vi "Digital_Input_32Channels.vi"(1 "IO":T1={"DI 0"="Mod1/DIO2", "DI 1"="Mod1/DIO2", "DI 2"="Mod1/DIO2", "DI 3"="Mod1/DIO2", "DI 4"="Mod1/DIO2", "DI 5"="Mod1/DIO2", "DI 6"="Mod1/DIO2", "DI 7"="Mod1/DIO2", "DI 8"="Mod1/DIO2", "DI 9"="Mod1/DIO2", "DI 10"="Mod1/DIO2", "DI 11"="Mod1/DIO2", "DI 12"="Mod1/DIO2", "DI 13"="Mod1/DIO2", "DI 14"="Mod1/DIO2", "DI 15"="Mod1/DIO2", "DI 16"="Mod1/DIO2", "DI 17"="Mod1/DIO2", "DI 18"="Mod1/DIO2", "DI 19"="Mod1/DIO2", "DI 20"="Mod1/DIO2", "DI 21"="Mod1/DIO2", "DI 22"="Mod1/DIO2", "DI 23"="Mod1/DIO2", "DI 24"="Mod1/DIO2", "DI 25"="Mod1/DIO2", "DI 26"="Mod1/DIO2", "DI 27"="Mod1/DIO2", "DI 28"="Mod1/DIO2", "DI 29"="Mod1/DIO2", "DI 30"="Mod1/DIO2", "DI 31"="Mod1/DIO2"}) -> (0 "States":bool[](array[boolean]))   [LabVIEW 2019, in "FPGA Wizard Templates.lvlib"]
uses:
  FPGA Wizard Templates.lvlib
  <vilib>/eio/EIONode/EIONode.xnode
  <vilib>/rvi/eio/common/nirviEmuTemplateMethod_errors.vi
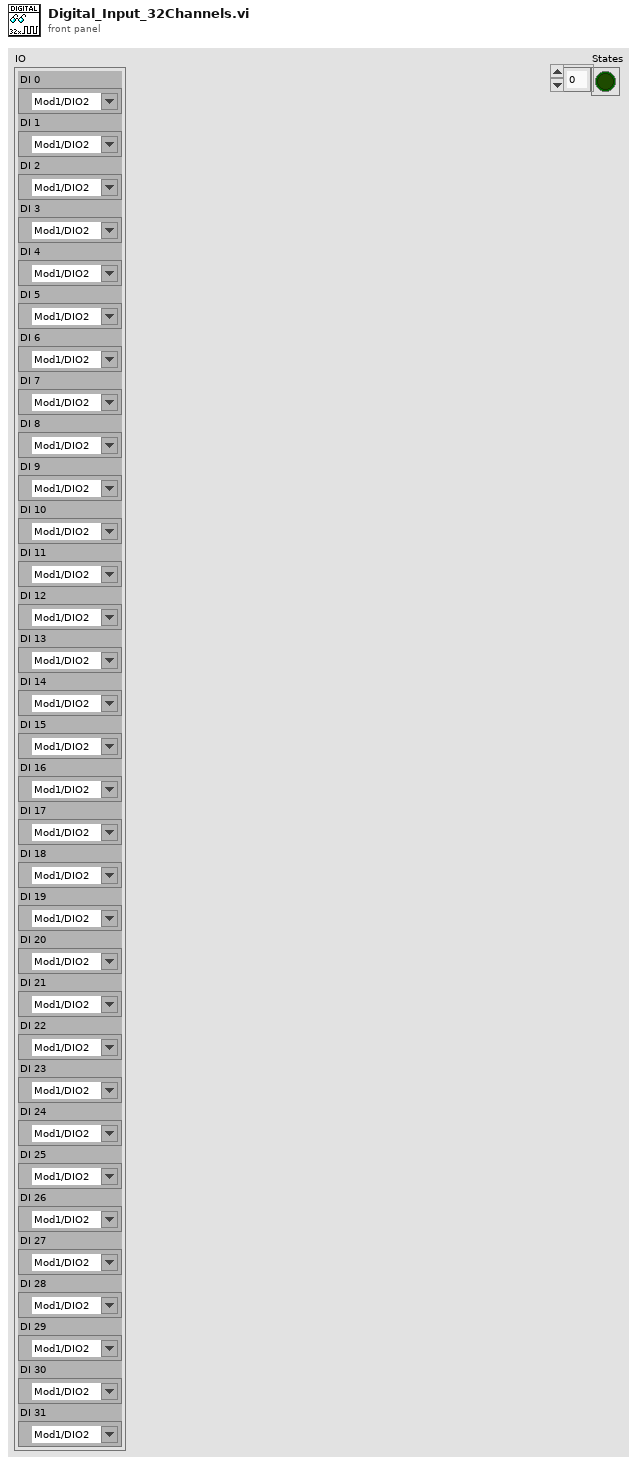
[diagram p1: front panel]
types:
  T1 = cluster{"DI 0":refnum<k21>, "DI 1":refnum<k21>, "DI 2":refnum<k21>, "DI 3":refnum<k21>, "DI 4":refnum<k21>, "DI 5":refnum<k21>, "DI 6":refnum<k21>, "DI 7":refnum<k21>, "DI 8":refnum<k21>, "DI 9":refnum<k21>, "DI 10":refnum<k21>, "DI 11":refnum<k21>, "DI 12":refnum<k21>, "DI 13":refnum<k21>, "DI 14":refnum<k21>, "DI 15":refnum<k21>, "DI 16":refnum<k21>, "DI 17":refnum<k21>, "DI 18":refnum<k21>, "DI 19":refnum<k21>, "DI 20":refnum<k21>, "DI 21":refnum<k21>, "DI 22":refnum<k21>, "DI 23":refnum<k21>, "DI 24":refnum<k21>, "DI 25":refnum<k21>, "DI 26":refnum<k21>, "DI 27":refnum<k21>, "DI 28":refnum<k21>, "DI 29":refnum<k21>, "DI 30":refnum<k21>, "DI 31":refnum<k21>}
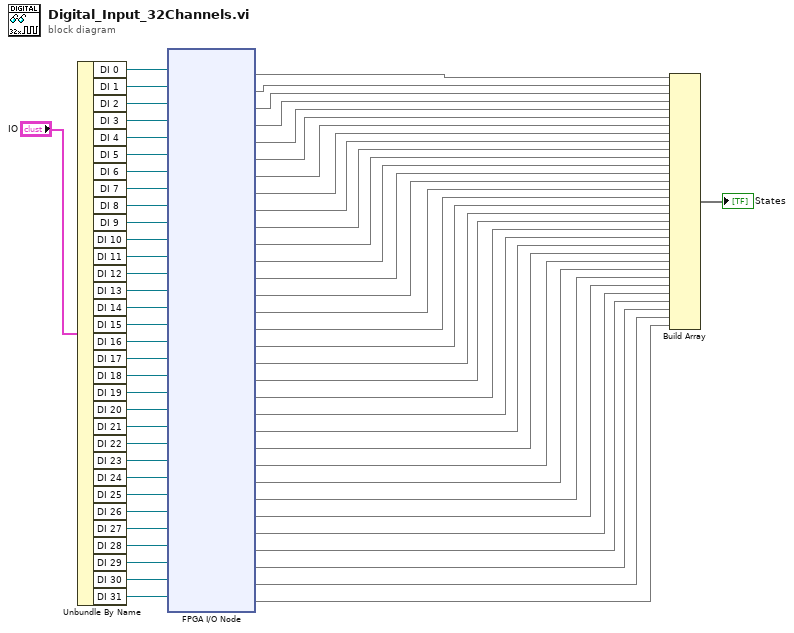
[diagram p0: block diagram]
diagram:
  n1 = Unbundle By Name("IO") -> ("DI 0"=w65:refnum<k21>, "DI 1"=w64:refnum<k21>, "DI 2"=w63:refnum<k21>, "DI 3"=w62:refnum<k21>, "DI 4"=w61:refnum<k21>, "DI 5"=w60:refnum<k21>, "DI 6"=w59:refnum<k21>, "DI 7"=w58:refnum<k21>, "DI 8"=w48:refnum<k21>, "DI 9"=w47:refnum<k21>, "DI 10"=w46:refnum<k21>, "DI 11"=w45:refnum<k21>, "DI 12"=w44:refnum<k21>, "DI 13"=w43:refnum<k21>, "DI 14"=w42:refnum<k21>, "DI 15"=w41:refnum<k21>, "DI 16"=w40:refnum<k21>, "DI 17"=w39:refnum<k21>, "DI 18"=w38:refnum<k21>, "DI 19"=w37:refnum<k21>, "DI 20"=w36:refnum<k21>, "DI 21"=w35:refnum<k21>, "DI 22"=w34:refnum<k21>, "DI 23"=w33:refnum<k21>, "DI 24"=w32:refnum<k21>, "DI 25"=w31:refnum<k21>, "DI 26"=w30:refnum<k21>, "DI 27"=w29:refnum<k21>, "DI 28"=w28:refnum<k21>, "DI 29"=w27:refnum<k21>, "DI 30"=w26:refnum<k21>, "DI 31"=w25:refnum<k21>)
  n2 = xnode "FPGA I/O Node"("FPGA I/O In"=w65, "FPGA I/O In"=w64, "FPGA I/O In"=w63, "FPGA I/O In"=w62, "FPGA I/O In"=w61, "FPGA I/O In"=w60, "FPGA I/O In"=w59, "FPGA I/O In"=w58, "FPGA I/O In"=w48, "FPGA I/O In"=w47, "FPGA I/O In"=w46, "FPGA I/O In"=w45, "FPGA I/O In"=w44, "FPGA I/O In"=w43, "FPGA I/O In"=w42, "FPGA I/O In"=w41, "FPGA I/O In"=w40, "FPGA I/O In"=w39, "FPGA I/O In"=w38, "FPGA I/O In"=w37, "FPGA I/O In"=w36, "FPGA I/O In"=w35, "FPGA I/O In"=w34, "FPGA I/O In"=w33, "FPGA I/O In"=w32, "FPGA I/O In"=w31, "FPGA I/O In"=w30, "FPGA I/O In"=w29, "FPGA I/O In"=w28, "FPGA I/O In"=w27, "FPGA I/O In"=w26, "FPGA I/O In"=w25) -> ("I/O Item"=w57, "I/O Item"=w56, "I/O Item"=w55, "I/O Item"=w54, "I/O Item"=w53, "I/O Item"=w52, "I/O Item"=w51, "I/O Item"=w50, "I/O Item"=w24, "I/O Item"=w23, "I/O Item"=w22, "I/O Item"=w21, "I/O Item"=w20, "I/O Item"=w19, "I/O Item"=w18, "I/O Item"=w17, "I/O Item"=w16, "I/O Item"=w15, "I/O Item"=w14, "I/O Item"=w13, "I/O Item"=w12, "I/O Item"=w11, "I/O Item"=w10, "I/O Item"=w9, "I/O Item"=w8, "I/O Item"=w7, "I/O Item"=w6, "I/O Item"=w5, "I/O Item"=w4, "I/O Item"=w3, "I/O Item"=w2, "I/O Item"=w1)  [unwired: 32 out]
  n3 = Build Array(w57, w56, w55, w54, w53, w52, w51, w50, w24, w23, w22, w21, w20, w19, w18, w17, w16, w15, w14, w13, w12, w11, w10, w9, w8, w7, w6, w5, w4, w3, w2, w1) -> (→"States":void[])
